vi "Read Events.vi"(8 "error in (no error)":errorcluster, 11 "Editor Handler in":refnum<class "Image Editor Handler.lvclass">) -> (0 "error out":errorcluster, 2 "Editor Events":T1, 3 "Editor Handler out":refnum<class "Image Editor Handler.lvclass">)   [LabVIEW 2015, in "LV Image Editor Framework.lvlib" / "Image Editor Handler.lvclass"]
uses:
  Image Editor Handler.lvclass
  Editor Events.ctl
  <vilib>/event_ctls.llb/eventvkey.ctl
  <vilib>/Utility/miscctls.llb/LVPoint32TypeDef.ctl
  Forms/Shape/Shape.lvclass
  Image Editor Handler.lvclass/Image Editor Handler.ctl
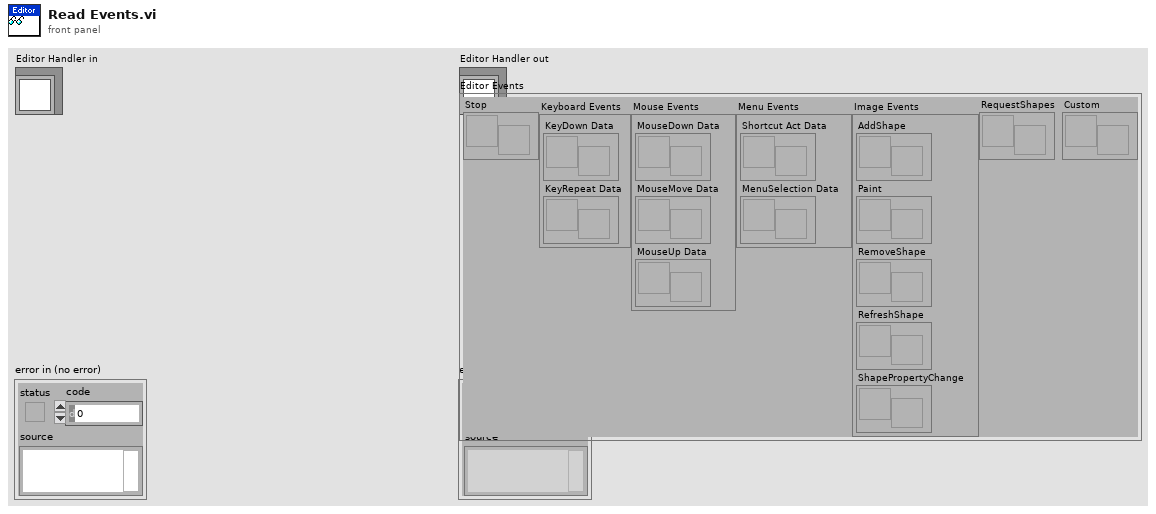
[diagram p1: front panel]
types:
  T1 = typedef "LV Image Editor Framework.lvlib/Image Editor Handler.lvclass/Editor Events.ctl" = cluster{"Stop":refnum<user-event>, "Keyboard Events":cluster{"KeyDown Data":refnum<user-event>, "KeyRepeat Data":refnum<user-event>}, "Mouse Events":cluster{"MouseDown Data":refnum<user-event>, "MouseMove Data":refnum<user-event>, "MouseUp Data":refnum<user-event>}, "Menu Events":cluster{"Shortcut Act Data":refnum<user-event>, "MenuSelection Data":refnum<user-event>}, "Image Events":cluster{"AddShape":refnum<user-event>, "Paint":refnum<user-event>, "RemoveShape":refnum<user-event>, "RefreshShape":refnum<user-event>, "ShapePropertyChange":refnum<user-event>}, "RequestShapes":refnum<user-event>, "Custom":refnum<user-event>}
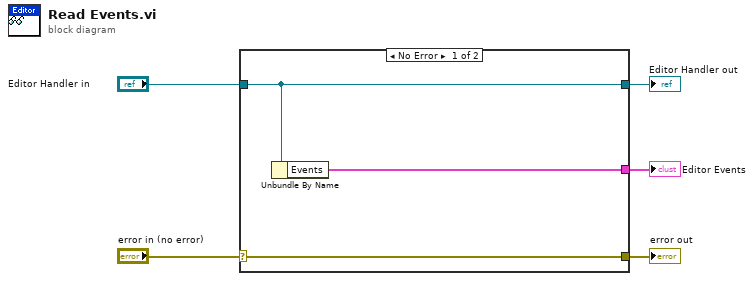
[diagram p0: block diagram]
diagram:
  n1 = case shown="No Error" "error in (no error)" {
    selector: "error in (no error)" -> [w8 w9]
    tunnel: [w8 w9] -> w4
    tunnel: [w7 w10] -> w2
    tunnel: "Editor Handler in" -> [w7 w10]
    tunnel: [w6 _] -> w1
    frame No Error {
      n2 = Unbundle By Name(w7) -> ("Events"=w6:T1)
    }
    frame Error {
    }
  }
  "error out" <- w4
  "Editor Handler out" <- w2
  "Editor Events" <- w1
